vi "Clear Hardware.vi"(2 "error in (no error)":errorcluster, 3 "DMD in":refnum<class "DMD.lvclass">) -> (0 "error out":errorcluster, 1 "DMD out":refnum<class "DMD.lvclass">)   [LabVIEW 2013, in "DMD.lvclass"]
doc: "This VI resets any necessary hardware so that the device will be ready for the next run."
uses:
  DMD.lvclass
  DMD.lvclass/DMD.ctl
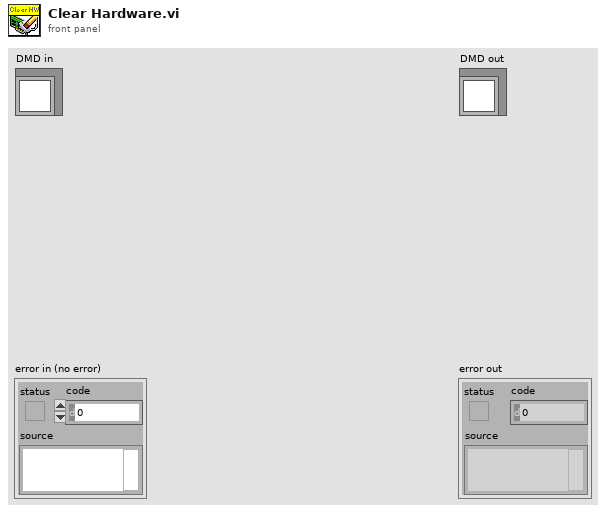
[diagram p1: front panel]
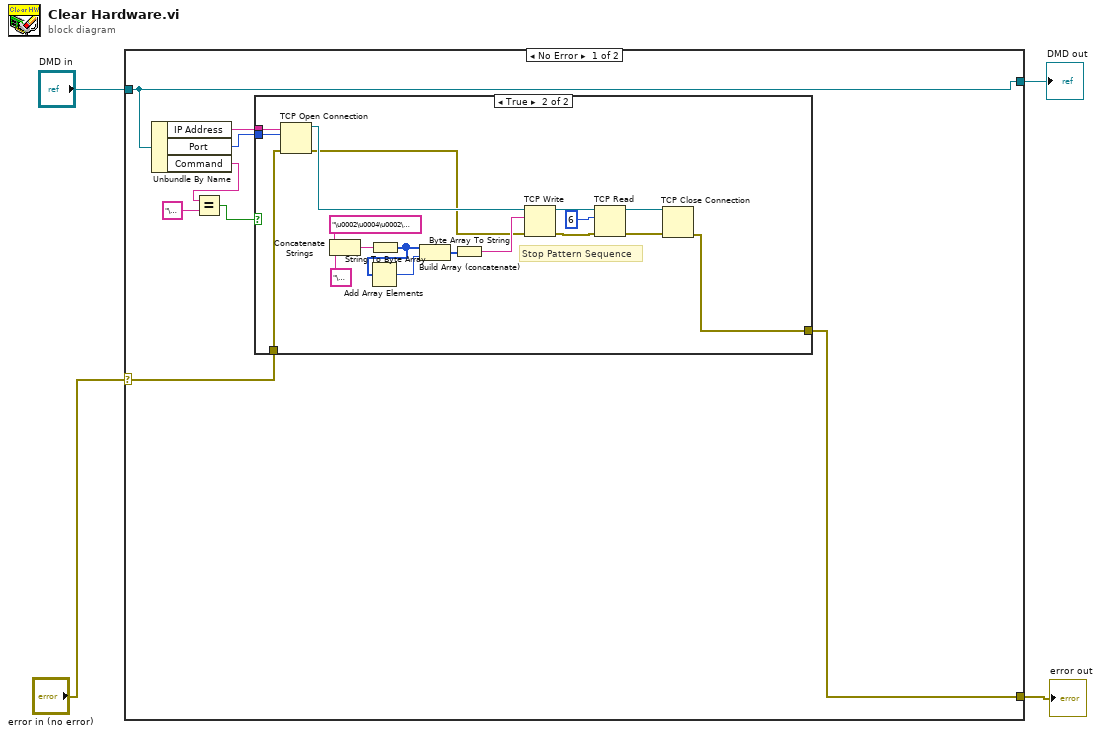
[diagram p0: block diagram]
diagram:
  n1 = case shown="No Error" "error in (no error)" {
    selector: "error in (no error)" -> [w10 w32]
    tunnel: "DMD in" -> [w6 w33]
    tunnel: [w6 w33] -> w3
    tunnel: [w5 w32] -> w2
    frame No Error {
      n2 = Unbundle By Name(w6) -> ("IP Address"=w12:string, "Port"=w11:u16, "Command"=w9:string)
      n3 = Equal?(x=w9, y="\u0004") -> (x = y?=w7:bool)
      n4 = case shown="True" w7 {
        tunnel: w12 -> [_ w31]
        tunnel: w11 -> [_ w30]
        tunnel: w10 -> [w13 w29]
        tunnel: [w13 w14] -> w5
        frame False {
        }
        frame True {
          # "Stop Pattern Sequence"
          n5 = TCP Open Connection(address=w31, remote port or service name=w30, error in (no error)=w29) -> (connection ID=w18:refnum<k5>, error out=w17:errorcluster)  [unwired: 2 in]
          n6 = Concatenate Strings("\u0002\u0004\u0002\u0000\u0001\u0000" ("string"), "\u0000" ("string")) -> (w24:string)
          n7 = String To Byte Array(string=w24) -> (unsigned byte array=w25:u8[])
          n8 = Add Array Elements(numeric array=w25) -> (sum=w26:u8)
          n9 = Build Array (concatenate)(w25, w26) -> (w27:u8[])
          n10 = Byte Array To String(unsigned byte array=w27) -> (string=w28:string)
          n11 = TCP Write(connection ID=w18, data in=w28, error in (no error)=w17) -> (connection ID out=w19:refnum<k5>, error out=w21:errorcluster)  [unwired: 1 in, 1 out]
          n12 = TCP Read(connection ID=w19, bytes to read=6, error in (no error)=w21) -> (connection ID out=w16:refnum<k5>, error out=w15:errorcluster)  [unwired: 2 in, 1 out]
          n13 = TCP Close Connection(connection ID=w16, error in (no error)=w15) -> (error out=w14:errorcluster)  [unwired: 1 in, 1 out]
        }
      }
    }
    frame Error {
    }
  }
  "error out" <- w2
  "DMD out" <- w3
